vi "Keithley 6517 Acquire Measurement.vi"() -> ()   [LabVIEW 2020]
doc: "This example shows how to acquire measurement data.\n\n\n<B>Note:</B>\nThis Example is compatible with both model 6517 and 6514."
uses:
  <instrlib>/Keithley 6517/Keithley 6517.lvlib
panel:
  in  "Enable Zero Correct (F: Disable)":bool
  in  "Instrument Model":i32(ring) items=["MODEL 6517B", "MODEL 6517A", "MODEL 6514"]
  in  "Reading Option (0: Latest)":i32(ring) items=["Latest", "New"]
  out "Measurement":T1 {"Measurement" format="%.6e"}
  in  "Enable Average Filter (F: Disable)":bool
  in  "Filter Count (10)":i32=10
  in  "Display Resolution (6)":dbl=6.0
  in  "Auto Range Value (2.0000000E+2)":dbl=200.0 format="%.7e"
  in  "Aperture Integration Time (1.6667000000E-2 s)":dbl=0.016667 format="%.10e"
  in  "Measurement Function (0: Voltage)":i32(ring) items=["Voltage", "Current", "Resistance", "Charge"]
  in  "VISA resource name":refnum<visa-resource-name>
  # "(c) 2016-2017 National Instruments.  ALL RIGHTS RESERVED."
  # "Note: This Example is compatible with model 6517 and 6514."
  # "6517 Only"
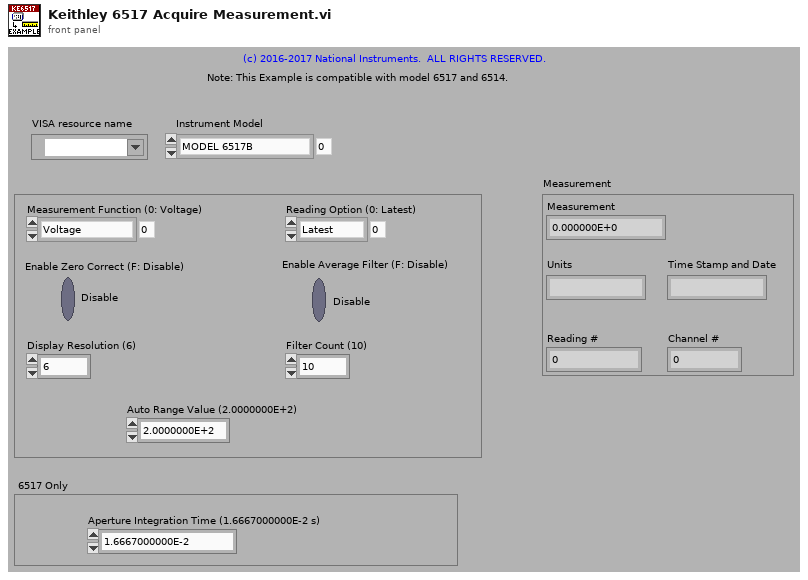
[diagram p1: front panel]
types:
  T1 = cluster{"Measurement":dbl, "Units":string, "Time Stamp and Date":string, "Reading #":dbl, "Channel #":dbl}
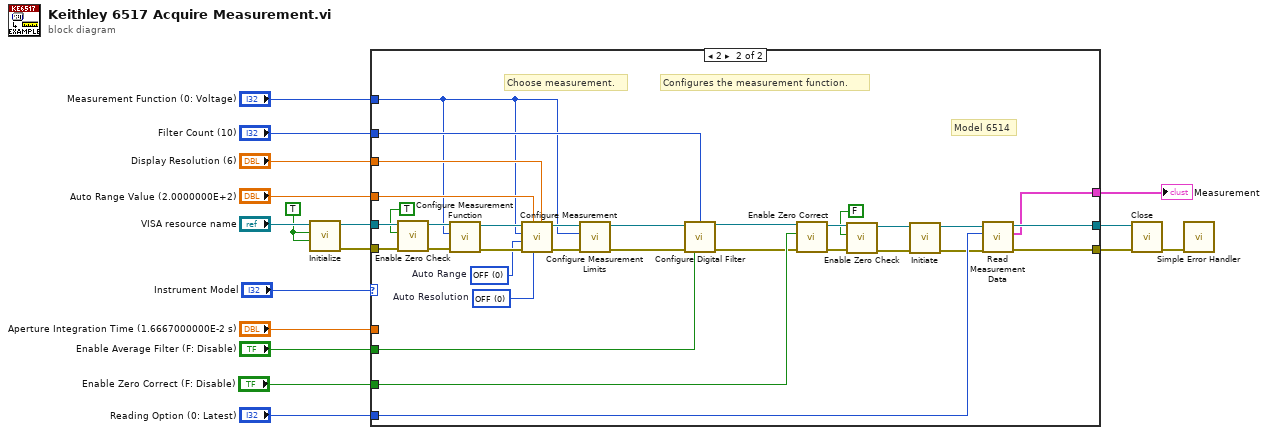
[diagram p0: block diagram]
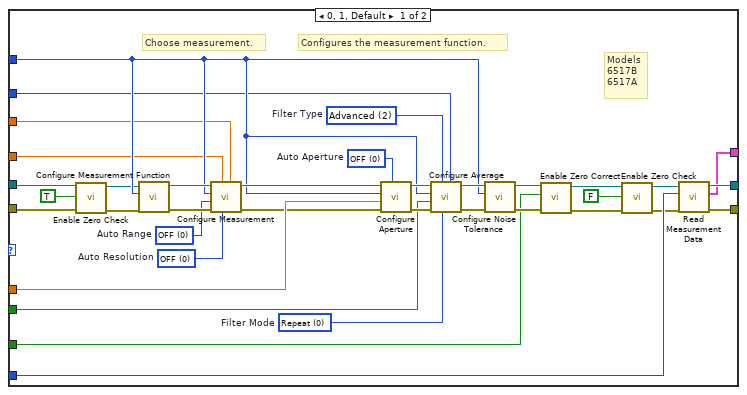
[diagram p2: hidden frame]
diagram:
  w7 = TRUE ("ID Query (True)")
  n1 = call <instrlib>:"Initialize.vi"("Reset (True)"=w7, "ID Query (True)"=w7, "VISA resource name"="VISA resource name") -> ("error out"=w4:errorcluster, "VISA resource name out"=w3:refnum<visa-resource-name>)  [unwired: 7 in]
  n2 = case shown="2" "Instrument Model" {
    tunnel: [w49 w85] -> w15
    tunnel: [w48 w84] -> w14
    tunnel: "Aperture Integration Time (1.6667000000E-2 s)" -> [w47 _]
    tunnel: "Measurement Function (0: Voltage)" -> [w42 w64]
    tunnel: "Auto Range Value (2.0000000E+2)" -> [w41 w81]
    tunnel: "Display Resolution (6)" -> [w40 w80]
    tunnel: "Filter Count (10)" -> [w38 w73]
    tunnel: "Enable Average Filter (F: Disable)" -> [w36 w74]
    tunnel: [w23 w60] -> w6
    tunnel: "Reading Option (0: Latest)" -> [w32 w77]
    tunnel: w4 -> [w25 w72]
    tunnel: w3 -> [w24 w71]
    tunnel: "Enable Zero Correct (F: Disable)" -> [w18 w63]
    frame 0, 1, Default {
      w33 = 0 items=["OFF", "ON", "ONCE"]  # Auto Aperture
      w34 = 0 items=["OFF", "ON", "ONCE"]  # Auto Resolution
      w39 = 2 items=["None", "Scalar", "Advanced"]  # Filter Type
      w37 = 0 items=["Repeat", "Moving"]  # Filter Mode
      w35 = 0 items=["OFF", "ON", "ONCE"]  # Auto Range
      # "Models\n6517B\n6517A"
      # "Choose measurement."
      # "Configures the measurement function."
      n3 = call <instrlib>:"Enable Zero Check.vi"("error in (no error)"=w25, "Enable Zero Check (T: Enable)"=TRUE ("Enable Zero Correct (F: Disable)"), "VISA resource name"=w24) -> ("error out"=w27:errorcluster, "VISA resource name out"=w26:refnum<visa-resource-name>)  [unwired: 7 in]
      n4 = call <instrlib>:"Configure Measurement Function.vi"("error in (no error)"=w27, "Measurement Function (0: Voltage)"=w42, "VISA resource name"=w26) -> ("error out"=w45:errorcluster, "VISA resource name out"=w46:refnum<visa-resource-name>)  [unwired: 7 in]
      n5 = call <instrlib>:"Configure Measurement.vi"("Display Resolution (6)"=w40, "Auto Resolution (1: ON)"=w34, "Auto Range Value (2.0000000E+2)"=w41, "error in (no error)"=w45, "Auto Range (1: ON)"=w35, "Measurement Function (0: Voltage)"=w42, "VISA resource name"=w46) -> ("error out"=w43:errorcluster, "VISA resource name out"=w44:refnum<visa-resource-name>)  [unwired: 3 in]
      n6 = call <instrlib>:"Configure Aperture.vi"("Auto Aperture (0: OFF)"=w33, "error in (no error)"=w43, "Aperture Integration Time (1.6667000000E-2 s)"=w47, "Measurement Function (0: Voltage)"=w42, "VISA resource name"=w44) -> ("error out"=w50:errorcluster, "VISA resource name out"=w51:refnum<visa-resource-name>)  [unwired: 5 in]
      n7 = call <instrlib>:"Configure Average.vi"("Filter Count (10)"=w38, "Filter Mode (0: Repeat)"=w37, "Filter Type (1: Scalar)"=w39, "error in (no error)"=w50, "Enable Average Filter (F: Disable)"=w36, "Measurement Function (0: Voltage)"=w42, "VISA resource name"=w51) -> ("error out"=w53:errorcluster, "VISA resource name out"=w52:refnum<visa-resource-name>)  [unwired: 3 in]
      n8 = call <instrlib>:"Configure Noise Tolerance.vi"("error in (no error)"=w53, "Measurement Function (0: Voltage)"=w42, "VISA resource name"=w52) -> ("error out"=w20:errorcluster, "VISA resource name out"=w19:refnum<visa-resource-name>)  [unwired: 7 in]
      n9 = call <instrlib>:"Enable Zero Correct.vi"("error in (no error)"=w20, "Enable Zero Correct (F: Disable)"=w18, "VISA resource name"=w19) -> ("error out"=w22:errorcluster, "VISA resource name out"=w21:refnum<visa-resource-name>)  [unwired: 7 in]
      n10 = call <instrlib>:"Enable Zero Check.vi"("error in (no error)"=w22, "Enable Zero Check (T: Enable)"=FALSE ("Enable Zero Correct (F: Disable)"), "VISA resource name"=w21) -> ("error out"=w31:errorcluster, "VISA resource name out"=w30:refnum<visa-resource-name>)  [unwired: 7 in]
      n11 = call <instrlib>:"Read Measurement Data.vi"("error in (no error)"=w31, "Reading Option (0: Latest)"=w32, "VISA resource name"=w30) -> ("error out"=w48:errorcluster, "Measurement"=w23:T1, "VISA resource name out"=w49:refnum<visa-resource-name>)  [unwired: 6 in]
    }
    frame 2 {
      w78 = 0 items=["OFF", "ON", "ONCE"]  # Auto Resolution
      w79 = 0 items=["OFF", "ON", "ONCE"]  # Auto Range
      # "Model 6514"
      # "Choose measurement."
      # "Configures the measurement function."
      n12 = call <instrlib>:"Enable Zero Check.vi"("error in (no error)"=w72, "Enable Zero Check (T: Enable)"=TRUE ("Enable Guard (F: Disable)"), "VISA resource name"=w71) -> ("error out"=w70:errorcluster, "VISA resource name out"=w69:refnum<visa-resource-name>)  [unwired: 7 in]
      n13 = call <instrlib>:"Configure Measurement Function.vi"("error in (no error)"=w70, "Measurement Function (0: Voltage)"=w64, "VISA resource name"=w69) -> ("error out"=w82:errorcluster, "VISA resource name out"=w83:refnum<visa-resource-name>)  [unwired: 7 in]
      n14 = call <instrlib>:"Configure Measurement.vi"("Display Resolution (6)"=w80, "Auto Resolution (1: ON)"=w78, "Auto Range Value (2.0000000E+2)"=w81, "error in (no error)"=w82, "Auto Range (1: ON)"=w79, "Measurement Function (0: Voltage)"=w64, "VISA resource name"=w83) -> ("error out"=w76:errorcluster, "VISA resource name out"=w75:refnum<visa-resource-name>)  [unwired: 3 in]
      n15 = call <instrlib>:"Configure Measurement Limits.vi"("error in (no error)"=w76, "Measurement Function (0: Voltage)"=w64, "VISA resource name"=w75) -> ("error out"=w59:errorcluster, "VISA resource name out"=w58:refnum<visa-resource-name>)  [unwired: 7 in]
      n16 = call <instrlib>:"Configure Digital Filter.vi"("VISA resource name"=w58, "Enable Digital Filter (F: Disable)"=w74, "Filter Count (10)"=w73, "error in (no error)"=w59) -> ("VISA resource name out"=w61:refnum<visa-resource-name>, "error out"=w62:errorcluster)  [unwired: 10 in]
      n17 = call <instrlib>:"Enable Zero Correct.vi"("error in (no error)"=w62, "Enable Zero Correct (F: Disable)"=w63, "VISA resource name"=w61) -> ("error out"=w67:errorcluster, "VISA resource name out"=w66:refnum<visa-resource-name>)  [unwired: 7 in]
      n18 = call <instrlib>:"Enable Zero Check.vi"("error in (no error)"=w67, "Enable Zero Check (T: Enable)"=FALSE ("Enable Guard (F: Disable)"), "VISA resource name"=w66) -> ("error out"=w57:errorcluster, "VISA resource name out"=w54:refnum<visa-resource-name>)  [unwired: 7 in]
      n19 = call <instrlib>:"Initiate.vi"("error in (no error)"=w57, "VISA resource name"=w54) -> ("error out"=w56:errorcluster, "VISA resource name out"=w55:refnum<visa-resource-name>)  [unwired: 8 in]
      n20 = call <instrlib>:"Read Measurement Data.vi"("error in (no error)"=w56, "Reading Option (0: Latest)"=w77, "VISA resource name"=w55) -> ("error out"=w84:errorcluster, "Measurement"=w60:T1, "VISA resource name out"=w85:refnum<visa-resource-name>)  [unwired: 6 in]
    }
  }
  "Measurement" <- w6
  n21 = call <instrlib>:"Close.vi"("error in (no error)"=w14, "VISA resource name"=w15) -> ("error out"=w17:errorcluster)  [unwired: 9 in]
  n22 = call <vilib>:"Simple Error Handler.vi"("error in (no error)"=w17) -> ()  [unwired: 4 in, 5 out]
